vi "subFILEmainGLD.vi"(9 "String containing Filename":string caption="Participant Name (FirstLast)", 10 "String of Folder Names":string caption="Participant Name (FirstLast)", 11 "File Folder":path=path "C:/Users/rsKite/Desktop/FSR DATA") -> (0 "error out":errorcluster, 3 "refnum out":refnum<file>)   [LabVIEW 2019]
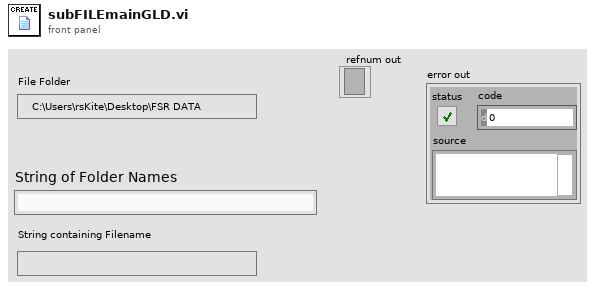
[diagram p1: front panel]
types:
  T1 = enum16{"open", "replace", "create", "open or create", "replace or create", "replace or create with confirmation"}
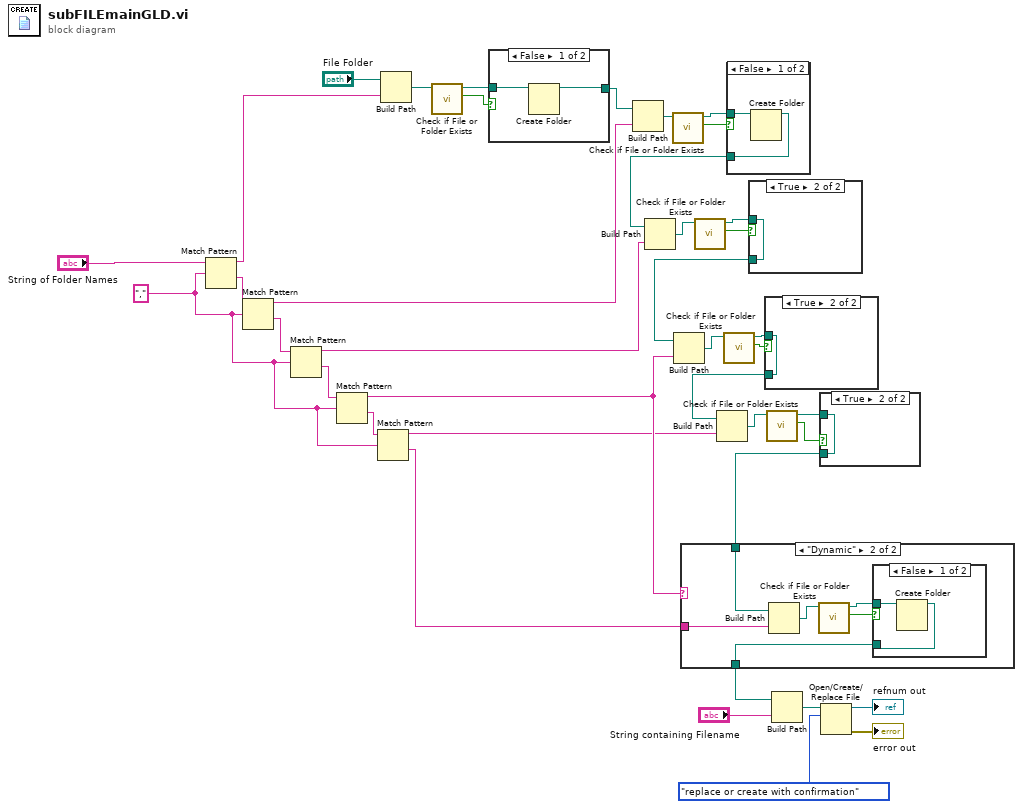
[diagram p0: block diagram]
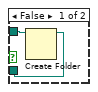
[diagram p2: hidden frame]
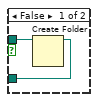
[diagram p5: hidden frame]
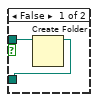
[diagram p6: hidden frame]
diagram:
  w27 = ","
  n1 = Match Pattern(string="String of Folder Names", regular expression=w27) -> (before substring=w13:string, after substring=w31:string)  [unwired: 1 in, 2 out]
  n2 = Match Pattern(string=w31, regular expression=w27) -> (before substring=w12:string, after substring=w29:string)  [unwired: 1 in, 2 out]
  n3 = Match Pattern(string=w29, regular expression=w27) -> (before substring=w10:string, after substring=w28:string)  [unwired: 1 in, 2 out]
  n4 = Match Pattern(string=w28, regular expression=w27) -> (before substring=w9:string, after substring=w26:string)  [unwired: 1 in, 2 out]
  n5 = Match Pattern(string=w26, regular expression=w27) -> (before substring=w5:string, after substring=w4:string)  [unwired: 1 in, 2 out]
  n6 = Build Path(base path="File Folder", name or relative path=w13) -> (appended path=w36:path)
  n7 = call <vilib>:"Check if File or Folder Exists.vi"("path"=w36) -> ("file or folder exists?"=w39:bool, "dup path"=w38:path)  [unwired: 8 in, 1 out]
  n8 = case shown="False" w39 {
    tunnel: w38 -> [w41 w42]
    tunnel: [w40 w42] -> w11
    frame False {
      n9 = Create Folder(path (use dialog)=w41) -> (created path=w40:path)  [unwired: 2 in, 2 out]
    }
    frame True {
    }
  }
  n10 = Build Path(base path=w11, name or relative path=w12) -> (appended path=w15:path)
  n11 = call <vilib>:"Check if File or Folder Exists.vi"("path"=w15) -> ("file or folder exists?"=w16:bool, "dup path"=w17:path)  [unwired: 8 in, 1 out]
  n12 = case shown="False" w16 {
    tunnel: w17 -> [w44 w45]
    tunnel: [w43 w45] -> w21
    frame False {
      n13 = Create Folder(path (use dialog)=w44) -> (created path=w43:path)  [unwired: 2 in, 2 out]
    }
    frame True {
    }
  }
  n14 = Build Path(base path=w21, name or relative path=w10) -> (appended path=w20:path)
  n15 = call <vilib>:"Check if File or Folder Exists.vi"("path"=w20) -> ("file or folder exists?"=w19:bool, "dup path"=w18:path)  [unwired: 8 in, 1 out]
  n16 = case shown="True" w19 {
    tunnel: w18 -> [w47 w48]
    tunnel: [w46 w48] -> w25
    frame False {
      n17 = Create Folder(path (use dialog)=w47) -> (created path=w46:path)  [unwired: 2 in, 2 out]
    }
    frame True {
    }
  }
  n18 = Build Path(base path=w25, name or relative path=w9) -> (appended path=w22:path)
  n19 = call <vilib>:"Check if File or Folder Exists.vi"("path"=w22) -> ("file or folder exists?"=w23:bool, "dup path"=w24:path)  [unwired: 8 in, 1 out]
  n20 = case shown="True" w23 {
    tunnel: w24 -> [w50 w51]
    tunnel: [w49 w51] -> w3
    frame False {
      n21 = Create Folder(path (use dialog)=w50) -> (created path=w49:path)  [unwired: 2 in, 2 out]
    }
    frame True {
    }
  }
  n22 = Build Path(base path=w3, name or relative path=w5) -> (appended path=w8:path)
  n23 = call <vilib>:"Check if File or Folder Exists.vi"("path"=w8) -> ("file or folder exists?"=w7:bool, "dup path"=w6:path)  [unwired: 8 in, 1 out]
  n24 = case shown="True" w7 {
    tunnel: w6 -> [w53 w54]
    tunnel: [w52 w54] -> w2
    frame False {
      n25 = Create Folder(path (use dialog)=w53) -> (created path=w52:path)  [unwired: 2 in, 2 out]
    }
    frame True {
    }
  }
  n26 = case shown="\"Dynamic\"" w9 {
    tunnel: w2 -> [w55 w58]
    tunnel: [w55 w57] -> w1
    tunnel: w4 -> [_ w56]
    frame "Static", Default {
    }
    frame "Dynamic" {
      n27 = Build Path(base path=w58, name or relative path=w56) -> (appended path=w59:path)
      n28 = call <vilib>:"Check if File or Folder Exists.vi"("path"=w59) -> ("file or folder exists?"=w60:bool, "dup path"=w61:path)  [unwired: 8 in, 1 out]
      n29 = case shown="False" w60 {
        tunnel: w61 -> [w63 w64]
        tunnel: [w62 w64] -> w57
        frame False {
          n30 = Create Folder(path (use dialog)=w63) -> (created path=w62:path)  [unwired: 2 in, 2 out]
        }
        frame True {
        }
      }
    }
  }
  n31 = Build Path(base path=w1, name or relative path="String containing Filename") -> (appended path=w34:path)
  n32 = Open/Create/Replace File(file path (use dialog)=w34, operation (0:open)=T1."replace or create with confirmation") -> (refnum out=→"refnum out":refnum<file>, error out=→"error out":errorcluster)  [unwired: 4 in, 1 out]
